vi "Lineup Log.vi"   [LabVIEW 2014]
uses:
  Begin/Global RefNums.vi
  <vilib>/Rock Robotics/WPI/Ultrasonic/WPI_SonarMB1010AnalogRefNum Registry Get.vi
  Begin/Global Variables.vi
  <vilib>/Rock Robotics/WPI/Ultrasonic/WPI_SonarMB1010AnalogGetRange.vi
types:
  T1 = typedef "WPI_SonarMB1010AnalogDeviceRef.ctl" = cluster{"AIDeviceRef":T2, "Scaling factor (V/in)":dbl, "Average Bits":u8}
  T2 = typedef "WPI_AnalogChannelDevRef.ctl" = cluster{"DevStatus":errorcluster, "Controller":T3, "Analog Channel":T4}
  T3 = typedef "FPGA_TypedefAnalogModule.ctl" = enum16{"Controller 1"}
  T4 = typedef "FPGA_AIChannel.ctl" = enum8{"AI 0", "AI 1", "AI 2", "AI 3", "AI MXP 0", "AI MXP 1", "AI MXP 2", "AI MXP 3", "Invalid"}
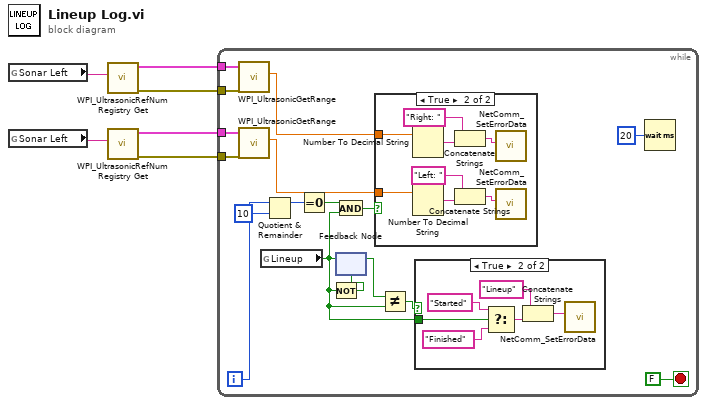
[diagram p0: block diagram]
diagram:
  n1 = global read "Global RefNums.vi" "Sonar Left"() -> (w1:string)
  n2 = global read "Global RefNums.vi" "Sonar Left"() -> (w6:string)
  n3 = call-poly <vilib>:"WPI_UltrasonicRefNum Registry Get.vi"("refnum name"=w1) -> ("error out"=w3:errorcluster, "SonarMB1010AnalogDevRef"=w2:T1)  [unwired: 9 in]
  n4 = call-poly <vilib>:"WPI_UltrasonicRefNum Registry Get.vi"("refnum name"=w6) -> ("error out"=w4:errorcluster, "SonarMB1010AnalogDevRef"=w5:T1)  [unwired: 9 in]
  n5 = while {
    tunnel: w5 -> [w23]
    tunnel: w4 -> [w22]
    tunnel: w2 -> [w8]
    tunnel: w3 -> [w9]
    i -> [w11]
    stop <- FALSE ("stop") stop-if-true
    n6 = call-poly <vilib>:"WPI_UltrasonicGetRange.vi"("error in"=w9, "SonarMB1010AnalogDevRef"=w8) -> ("Distance"=w7:dbl)  [unwired: 7 in, 2 out]
    n7 = call-poly <vilib>:"WPI_UltrasonicGetRange.vi"("error in"=w22, "SonarMB1010AnalogDevRef"=w23) -> ("Distance"=w21:dbl)  [unwired: 7 in, 2 out]
    n8 = global read "Global Variables.vi" "Lineup"() -> (w14:bool)
    n9 = Quotient & Remainder(x=w11, y=10) -> (x-y*floor(x/y)=w12:i32)  [unwired: 1 out]
    n10 = Equal To 0?(x=w12) -> (x = 0?=w13:bool)
    n11 = Not(x=w14) -> (.not. x?=w19:bool)
    n12 = And(x=w13, y=w14) -> (x .and. y?=w15:bool)
    n13 = feedback #1(w19) -> (w20:bool)
    n14 = feedback-in #1(w14) -> ()
    n15 = case shown="True" w15 {
      tunnel: w21 -> [_ w37]
      tunnel: w7 -> [_ w30]
      frame False {
      }
      frame True {
        n16 = Number To Decimal String(number=w30) -> (decimal integer string=w31:string)  [unwired: 1 in]
        n17 = Number To Decimal String(number=w37) -> (decimal integer string=w36:string)  [unwired: 1 in]
        n18 = Concatenate Strings("Right: " ("string"), w31) -> (w32:string)
        n19 = Concatenate Strings("Left: " ("string"), w36) -> (w35:string)
        n20 = call <vilib>:"NetComm_SetErrorData.vi"("Error Data"=w32) -> ()  [unwired: 3 in, 8 out]
        n21 = call <vilib>:"NetComm_SetErrorData.vi"("Error Data"=w35) -> ()  [unwired: 3 in, 8 out]
      }
    }
    n22 = Not Equal?(x=w20, y=w14) -> (x != y?=w18:bool)
    n23 = case shown="True" w18 {
      tunnel: w14 -> [_ w29]
      frame False {
      }
      frame True {
        n24 = Select(t="Started" ("string"), s=w29, f="Finished" ("string")) -> (s? t:f=w26:string)
        n25 = Concatenate Strings("Lineup" ("string"), w26) -> (w25:string)
        n26 = call <vilib>:"NetComm_SetErrorData.vi"("Error Data"=w25) -> ()  [unwired: 3 in, 8 out]
      }
    }
    n27 = Wait (ms)(milliseconds to wait=u32 20) -> ()  [unwired: 1 out]
  }
